vi "Fcurve_GetAttributes.vi"(0 "reference in":refnum<class "Fcurve.lvclass">, 1 "return data? (T)":bool=TRUE, 5 "error in (no error)":errorcluster) -> (14 "reference out":refnum<class "Fcurve.lvclass">, 15 "attributes ref":T7, 16 "attributes":T1={"MyAttribute"=0.0, "Fcurve Metadata"={"dt (us)"=0.0, "Dec Factor"=0.0, "Z piezo Sensitivity (nm/V)"=0.0, "K (N/m)"=0.0, "Sp (V)"=0.0, "Contact (ms)"=0.0, "Zpos contact"=0.0, "Vel_app (nm/s)"=0.0, "Vel_ret (nm/s)"=0.0, "deltaV (nm)"=0.0, "Def_V0 (v)"=0.0, "Piezo gain"=0.0, "invOLS (nm/V)"=0.0}, "Contact Spread of dev"=2.0, "Tau Delay (ms)"=0.0, "Points of contact"=0.0, "Def_wfm"={"Max"=0.0, "Min"=0.0}, "Zpos_wfm"={"Max"=0.0, "Min"=0.0}, "Contact stat?"=FALSE, "Real AI dt (s)"=2.0, "Decimation"={"App"={"Dec"=2, "apply"=FALSE}, "Con"={"Dec"=1, "apply"=FALSE}, "Ret"={"Dec"=1, "apply"=FALSE}}, "Segment def[0]"=0.0, "Segment Zpos[0]"=0.0, "Raw Datum"=[], "Group metadata"={"property names"=[], "property values"=[]}, "M_data obj"=refnum, "Channel name(s)"=[], "Segment fcurve data"=[], "Segment duration"=[], "Segment info"=[], "Segment durations (S)"=[], "Segments Maxmin"=[]} {"Segment durations (S)" format="%0.2f"; "Real AI dt (s)" format="%#_13g"; "Tau Delay (ms)" format="%#_13g"; "Contact Spread of dev" format="%#_13g"}, 19 "error out":errorcluster)   [LabVIEW 2019, in "Fcurve.lvclass"]
doc: "Returns a reference and if wanted the actual data values of the attributes. This method is used by the subclasses to access parent attributes."
uses:
  Fcurve.lvclass
  C:/Program Files/National Instruments/LabVIEW 2019/vi.lib/addons/_AddQ/G#Object/G#Object.lvclass
  ObjectAttributesRef.ctl
  protected/ObjectAttributes.ctl
  Metadata.ctl
  TDMS_DataHandler_class/Fcurve Meta data.ctl
  metadata_class/metadata.lvclass
  Fcurve segments --cluster.ctl
  metadata_class/Segment type--combobox.ctl
  Segment MaxMin --cluster.ctl
  Fcurve.lvclass/Fcurve.ctl
  <vilib>/addons/_AddQ/G#Object/G#Object.lvclass
  TDMS_DataHandler_class/TDMS_DataHandler.lvclass
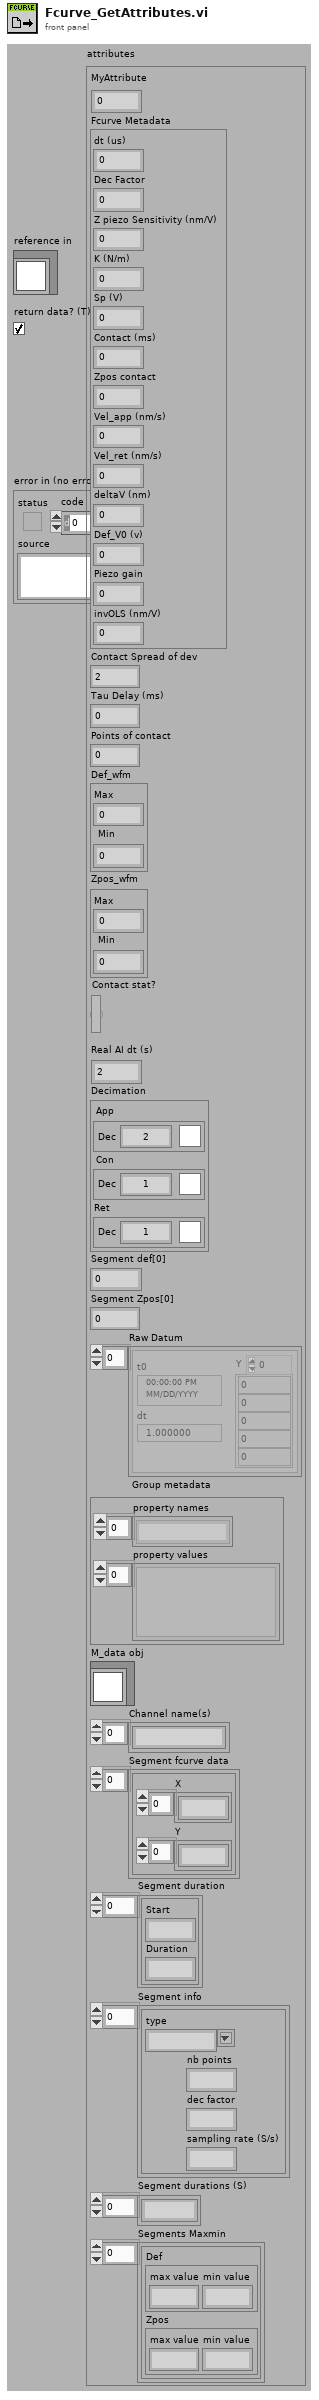
[diagram p1: front panel]
types:
  T1 = typedef "Fcurve.lvclass/ObjectAttributes.ctl" = cluster{"MyAttribute":dbl, "Fcurve Metadata":T2, "Contact Spread of dev":dbl, "Tau Delay (ms)":dbl, "Points of contact":dbl, "Def_wfm":cluster{"Max":dbl, "Min":dbl}, "Zpos_wfm":cluster{"Max":dbl, "Min":dbl}, "Contact stat?":bool, "Real AI dt (s)":dbl, "Decimation":cluster{"App":cluster{"Dec":i32, "apply":bool}, "Con":cluster{"Dec":i32, "apply":bool}, "Ret":cluster{"Dec":i32, "apply":bool}}, "Segment def[0]":dbl, "Segment Zpos[0]":dbl, "Raw Datum":waveform(dbl)[], "Group metadata":T3, "M_data obj":refnum<class "metadata.lvclass">, "Channel name(s)":string[], "Segment fcurve data":cluster{"X":dbl[], "Y":dbl[]}[], "Segment duration":cluster{"Start":i32, "Duration":i32}[], "Segment info":T4[], "Segment durations (S)":dbl[], "Segments Maxmin":T6[]}
  T2 = typedef "Fcurve.lvclass/Metadata.ctl" = cluster{"dt (us)":dbl, "Dec Factor":dbl, "Z piezo Sensitivity (nm/V)":dbl, "K (N/m)":dbl, "Sp (V)":dbl, "Contact (ms)":dbl, "Zpos contact":dbl, "Vel_app (nm/s)":dbl, "Vel_ret (nm/s)":dbl, "deltaV (nm)":dbl, "Def_V0 (v)":dbl, "Piezo gain":dbl, "invOLS (nm/V)":dbl}
  T3 = typedef "TDMS_DataHandler.lvclass/Fcurve Meta data.ctl" = cluster{"property names":string[], "property values":variant[]}
  T4 = typedef "Fcurve.lvclass/Fcurve segments --cluster.ctl" = cluster{"type":T5, "nb points":i32, "dec factor":u32, "sampling rate (S/s)":u32}
  T5 = typedef "metadata.lvclass/Segment type--combobox.ctl" = string
  T6 = typedef "Fcurve.lvclass/Segment MaxMin --cluster.ctl" = cluster{"Def":cluster{"max value":dbl, "min value":dbl}, "Zpos":cluster{"max value":dbl, "min value":dbl}}
  T7 = typedef "Fcurve.lvclass/ObjectAttributesRef.ctl" = refnum<data-value>
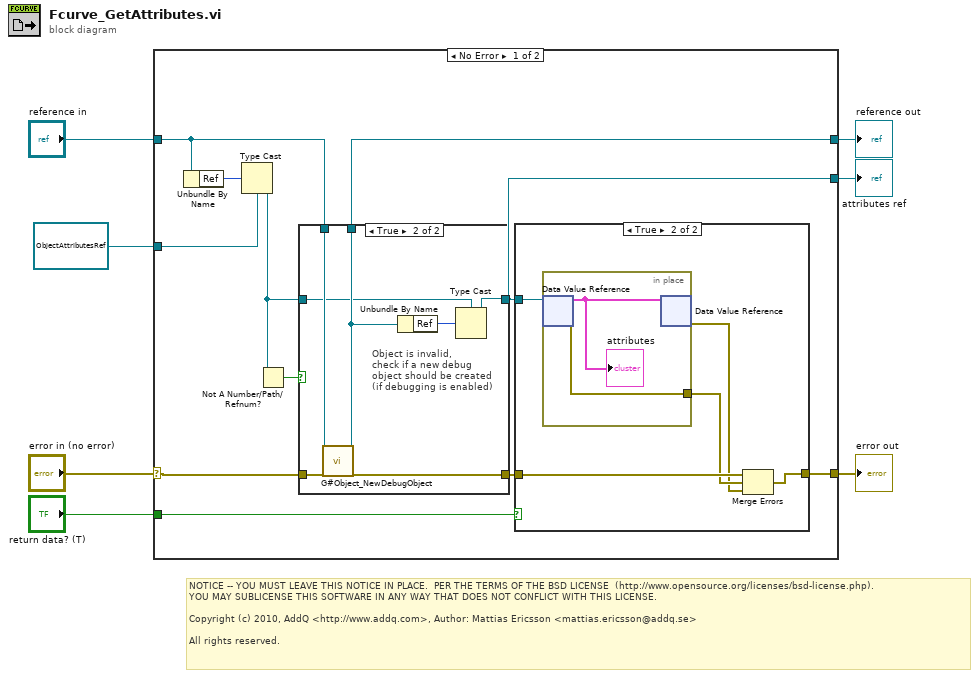
[diagram p0: block diagram]
diagram:
  # "NOTICE -- YOU MUST LEAVE THIS NOTICE IN PLACE.  PER THE TERMS OF THE BSD LICENSE  (http://www.opensource.org/licenses/bsd-license.php).\nYOU MAY SUBLICENSE THIS SOFTWARE IN ANY WAY THAT DOES NOT CONFLICT WITH THIS LICENSE.\n\nCopyright (c) 2010, AddQ <http://www.addq.com>, Author: Mattias Ericsson <mattias.ericsson@addq.se>\n\nAll rights reserved."
  n1 = case shown="No Error" "error in (no error)" {
    selector: "error in (no error)" -> [w14 w39]
    tunnel: [w17 w39] -> w6
    tunnel: [w11 w38] -> w4
    tunnel: "reference in" -> [w12 w38]
    tunnel: [w8 w37] -> w3
    tunnel: "return data? (T)" -> [w18 _]
    tunnel: T7 refnum ("attributes ref") -> [w10 w37]
    frame No Error {
      n2 = Unbundle By Name(w12) -> ("Ref"=w16:u32)
      n3 = Type Cast(type=w10, x=w16) -> (*(type *) &x=w9:T7)
      n4 = Not A Number/Path/Refnum?(number/path/refnum=w9) -> (NaN/Path/Refnum?=w13:bool)
      n5 = case shown="True" w13 {
        tunnel: [w21 w28] -> w15
        tunnel: w14 -> [w21 w27]
        tunnel: w12 -> [w20 w26]
        tunnel: [w20 w24] -> w11
        tunnel: w9 -> [w19 w23]
        tunnel: [w19 w22] -> w8
        frame False {
        }
        frame True {
          # "Object is invalid,\ncheck if a new debug\nobject should be created\n(if debugging is enabled)"
          n6 = call <vilib>:"G#Object_NewDebugObject.vi"("reference in"=w26, "error in (no error)"=w27) -> ("reference out"=w24:refnum<class "Fcurve.lvclass">, "error out"=w28:errorcluster)  [unwired: 16 in]
          n7 = Unbundle By Name(w24) -> ("Ref"=w25:u32)
          n8 = Type Cast(type=w23, x=w25) -> (*(type *) &x=w22:T7)
        }
      }
      n9 = case shown="True" w18 {
        tunnel: w8 -> [_ w34]
        tunnel: w15 -> [w29 w33]
        tunnel: [w29 w32] -> w17
        frame False {
        }
        frame True {
          n10 = in-place {
            in-place-border: [w36] -> w31
            n11 = in-place-dvr #1(w34) -> (w35:T1, w36:errorcluster)
            "attributes" <- w35
            n12 = in-place-dvr #1(w35) -> (w30:errorcluster)  [unwired: 1 out]
          }
          n13 = Merge Errors(w33, w31, w30) -> (w32:errorcluster)
        }
      }
    }
    frame Error {
    }
  }
  "error out" <- w6
  "reference out" <- w4
  "attributes ref" <- w3
